vi "Pre-Install Custom Action.vi"(10 "Variant":variant) -> (0 "error out":errorcluster)   [LabVIEW 2024]
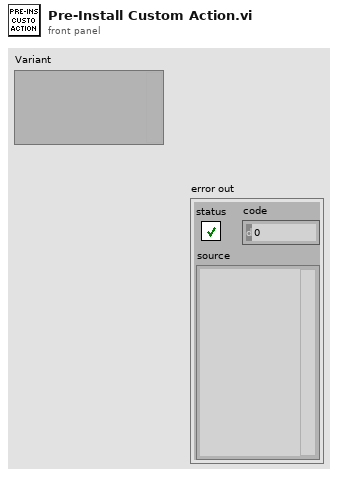
[diagram p1: front panel]
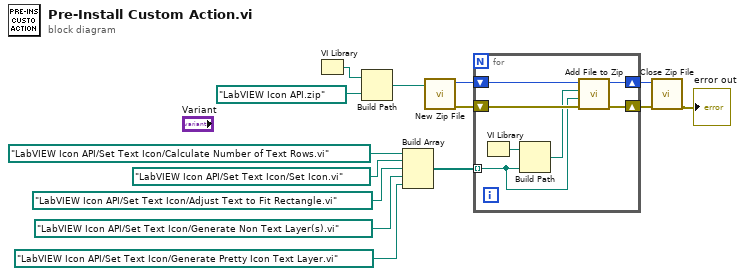
[diagram p0: block diagram]
diagram:
  n1 = VI Library() -> (path=w3:path)
  n2 = Build Path(base path=w3, name or relative path=path "LabVIEW Icon API.zip") -> (appended path=w8:path)
  n3 = Build Array(path "LabVIEW Icon API/Set Text Icon/Calculate Number of Text Rows.vi", path "LabVIEW Icon API/Set Text Icon/Set Icon.vi", path "LabVIEW Icon API/Set Text Icon/Adjust Text to Fit Rectangle.vi", path "LabVIEW Icon API/Set Text Icon/Generate Non Text Layer(s).vi", path "LabVIEW Icon API/Set Text Icon/Generate Pretty Icon Text Layer.vi") -> (w2:path[])
  n4 = call <vilib>:"New Zip File.vi"("target"=w8) -> ("error out"=w6:errorcluster, "zip file out"=w7:i64)  [unwired: 2 in, 3 out]
  n5 = for {
    shift-right: [w19] -> w5
    shift-left: w7 -> [w21]
    shift-right: [w18] -> w4
    shift-left: w6 -> [w20]
    tunnel: w2 -> [w15] mode=indexing
    n6 = VI Library() -> (path=w17:path)
    n7 = Build Path(base path=w17, name or relative path=w15) -> (appended path=w16:path)
    n8 = call <vilib>:"Add File to Zip.vi"("error in (no error)"=w20, "destination path in zip"=w15, "source file path"=w16, "zip file in"=w21) -> ("error out"=w18:errorcluster, "zip file out"=w19:i64)  [unwired: 6 out]
  }
  n9 = call <vilib>:"Close Zip File.vi"("error in (no error)"=w4, "zip file in"=w5) -> ("error out"=→"error out":errorcluster)  [unwired: 1 in, 4 out]
